vi "TEST_3KantVip.vi"() -> ()   [LabVIEW 2018]
panel:
  out "s? t:f":i32
  in  "stop":bool
  in  "BUND!":bool
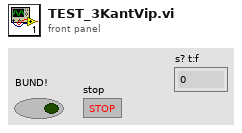
[diagram p1: front panel]
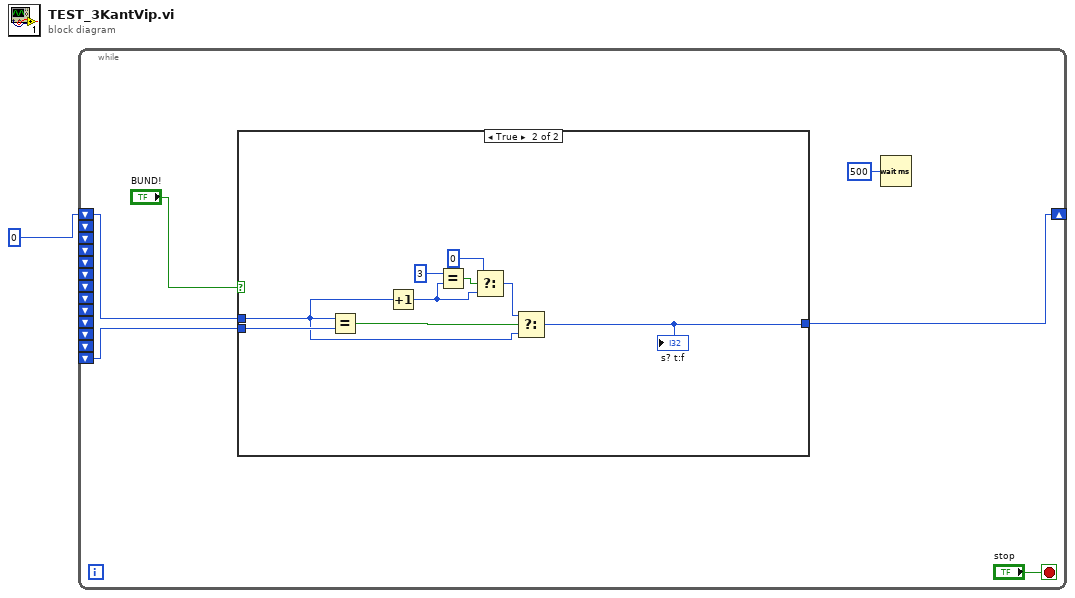
[diagram p0: block diagram]
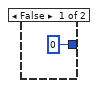
[diagram p2: hidden frame]
diagram:
  n1 = while {
    shift-right: [w3] -> _
    shift-left: 0 -> [w4]
    shift-left: _ -> [_]
    shift-left: _ -> [_]
    shift-left: _ -> [_]
    shift-left: _ -> [_]
    shift-left: _ -> [_]
    shift-left: _ -> [_]
    shift-left: _ -> [_]
    shift-left: _ -> [_]
    shift-left: _ -> [_]
    shift-left: _ -> [_]
    shift-left: _ -> [_]
    shift-left: _ -> [w5]
    stop <- "stop" stop-if-true
    n2 = case shown="True" "BUND!" {
      tunnel: w5 -> [_ w17]
      tunnel: w4 -> [_ w13]
      tunnel: [0 ("t") w9] -> w3
      frame False {
      }
      frame True {
        n3 = Equal?(x=w13, y=w17) -> (x = y?=w16:bool)
        n4 = Increment(x=w13) -> (x+1=w12:i32)
        n5 = Equal?(x=3, y=w12) -> (x = y?=w15:bool)
        n6 = Select(t=0, s=w15, f=w12) -> (s? t:f=w14:i32)
        n7 = Select(t=w14, s=w16, f=w13) -> (s? t:f=w9:i32)
        "s? t:f" <- w9
      }
    }
    n8 = Wait (ms)(milliseconds to wait=u32 500) -> ()  [unwired: 1 out]
  }
